vi "Store Rel Value.vi"(7 "Mode (T: Store)":bool=TRUE, 8 "Error In (no error)":errorcluster, 9 "Value Type (0: XY)":u16(ring) items=["XY", "R[dBm] Phi"], 10 "Scan Point (1)":i32=1, 11 "VISA Resource Name":refnum<visa-resource-name>) -> (0 "Error Out":errorcluster, 3 "VISA Resource Name Out":refnum<visa-resource-name>)   [LabVIEW 2010, in "Stanford Research 844.lvlib"]
doc: "This VI stores or clears the Rel Values along with the measurement configuration at the current frequency."
uses:
  <instrlib>/Stanford Research 844/Stanford Research 844.lvlib
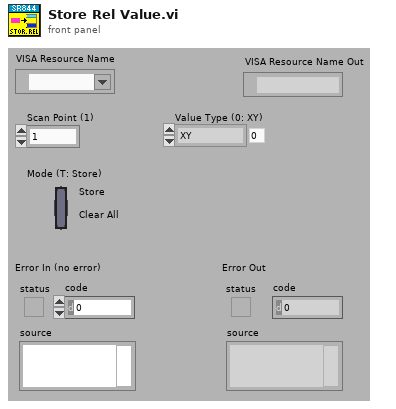
[diagram p1: front panel]
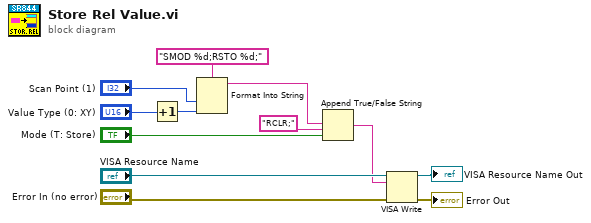
[diagram p0: block diagram]
diagram:
  n1 = Increment(x="Value Type (0: XY)") -> (x+1=w2:u16)
  n2 = Format Into String(format string="SMOD %d;RSTO %d;", "Scan Point (1)", w2) -> (resulting string=w5:string)  [unwired: 2 in, 1 out]
  n3 = Append True/False String(1:"Mode (T: Store)", 2:"RCLR;" ("true string"), 3:w5) -> (0:w1:string)  [unwired: 1 in]
  n4 = VISA Write(VISA resource name="VISA Resource Name", write buffer=w1, error in (no error)="Error In (no error)") -> (VISA resource name out=→"VISA Resource Name Out":refnum<visa-resource-name>, error out=→"Error Out":errorcluster)  [unwired: 1 out]
